vi "Set scroll bars ranges.vi"(8 "error in (no error)":errorcluster, 10 "Number of frames":u32) -> (0 "error out":errorcluster)   [LabVIEW 2020]
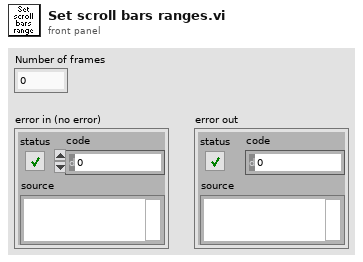
[diagram p1: front panel]
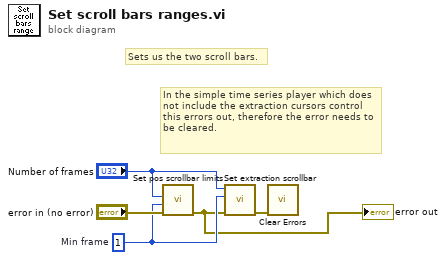
[diagram p0: block diagram]
diagram:
  w4 = u32 1  # Min frame
  # "In the simple time series player which does not include the extraction cursors control this errors out, therefore the error needs to be cleared."
  # "Sets us the two scroll bars."
  n1 = call "Set pos scrollbar limits.vi"("error in (no error)"="error in (no error)", "Min frame (unity-based)"=w4, "Max frame (unity-based)"="Number of frames") -> ("error out"=w2:errorcluster)  [unwired: 8 in]
  "error out" <- w2
  n2 = call "Set extraction scrollbar.vi"("error in (no error)"=w2, "Min frame"=w4, "Number of frames"="Number of frames") -> ("error out"=w1:errorcluster)  [unwired: 8 in]
  n3 = call <vilib>:"Clear Errors.vi"("error in (no error)"=w1) -> ()  [unwired: 5 in, 2 out]
